vi "Image_Acquire_simulate.vi"(0 "Queue Ref in":T3, 1 "Acquire Time":i32=100, 3 "Image Out":T2, 5 "error in (no error)":errorcluster, 7 "Test Timing":bool) -> (6 "Loop Time Out":i64, 8 "error out":errorcluster)   [LabVIEW 2019]
uses:
  <vilib>/vision/Image Controls.llb/IMAQ Image.ctl
  <vilib>/userDefined/High Color/IMAQdx.ctl
  <vilib>/Platform/TimedLoop/XDataNode/timing_clust.ctl
  <vilib>/Platform/TimedLoop/XDataNode/nitl_modes.ctl
  <vilib>/Platform/TimedLoop/XDataNode/wakeup.ctl
  <vilib>/Platform/TimedLoop/XDataNode/XDataNode.xnode
  <vilib>/Platform/TimedLoop/XDataNode/XDNodeRunTimeDep.lvlib
panel:
  in  "Session In":T1
  out "Global End Time":i64
  out "Iteration Duration":i64
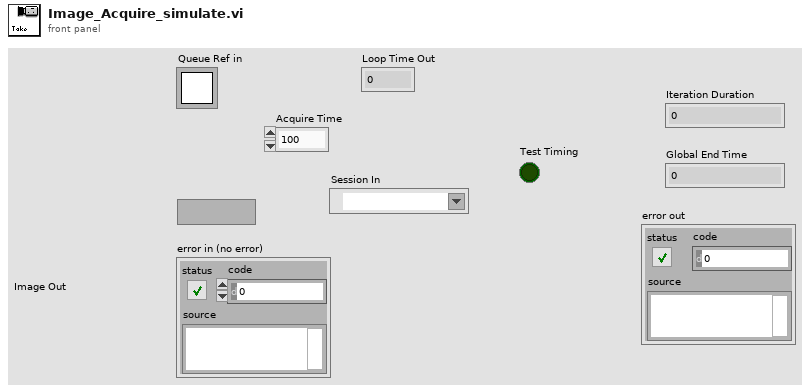
[diagram p1: front panel]
types:
  T1 = typedef "IMAQdx.ctl" = refnum<k21>
  T2 = typedef "IMAQ Image.ctl" = refnum<image>
  T3 = typedef "Queue RefNum" = refnum<k1>
  T4 = typedef "XDNodeRunTimeDep.lvlib/timing_clust.ctl" = cluster{"Expected End [f-1]":u64, "Actual End [f-1]":u64, "Finished Late? [f-1]":bool, "Expected End [i-1]":u64, "Actual End [i-1]":u64, "Finished Late? [i-1]":bool, "Expected Start [i]":u64, "Actual Start [i]":u64, "Expected Start [f]":u64, "Actual Start [f]":u64, "Source Name":string, "Structure Name":string, "Period":i64, "Deadline":i64, "Offset":i64, "Start":i64, "Priority":i32, "Timeout":i32, "Mode":T5, "Wakeup Reason":T6, "Error":errorcluster, "Source Type":string, "Secondary Source Type":string, "Global End Time":u64, "Global Start Time":u64, "Frame Duration":u64, "Iteration Duration":u64, "Assigned CPU":i32, "I/O Scan Engine Mode":u32}
  T5 = typedef "XDNodeRunTimeDep.lvlib/nitl_modes.ctl" = enum32{"No Change", "Process missed periods, maintain original phase", "Discard missed periods, maintain original phase", "Process missed periods, ignore original phase", "Discard missed periods, ignore original phase"}
  T6 = typedef "XDNodeRunTimeDep.lvlib/wakeup.ctl" = enum32{"Normal", "Aborted", "Asynchronous wakeup", "Timing source error", "Timed loop error", "Timeout"}
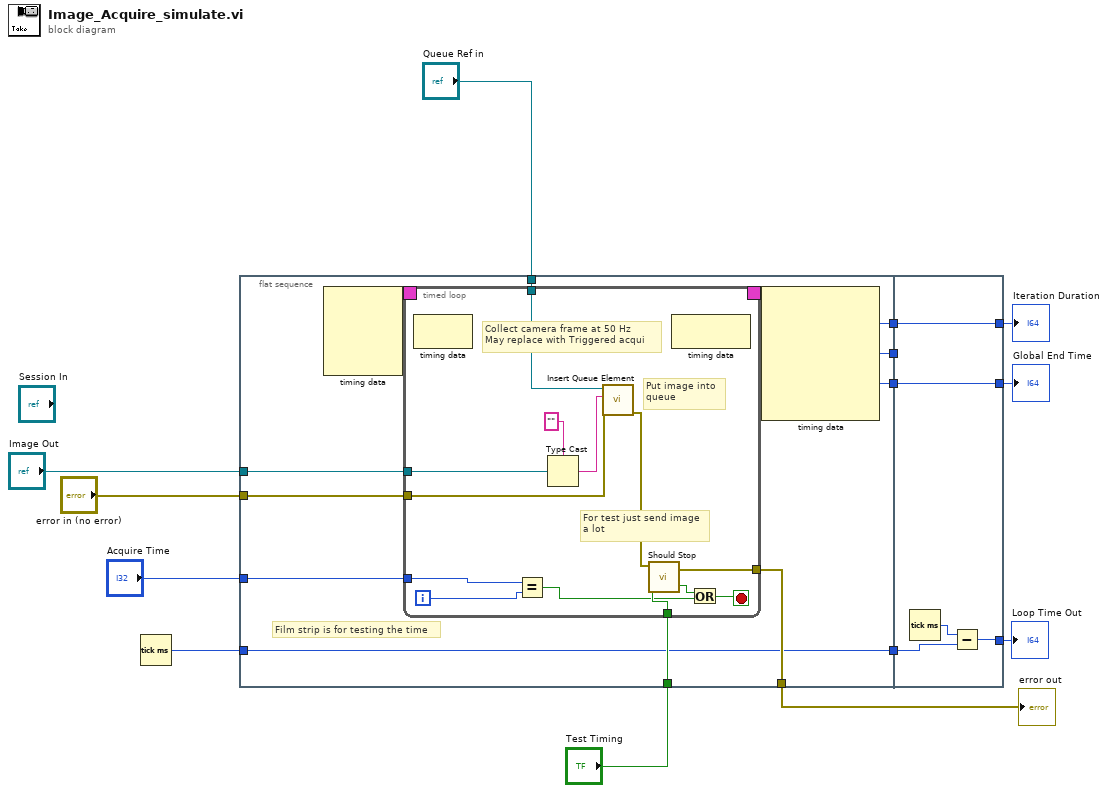
[diagram p0: block diagram]
diagram:
  n1 = Tick Count (ms)() -> (millisecond timer value=w1:u32)
  n2 = flat-sequence {
    tunnel: "error in (no error)" -> [w24]
    tunnel: "Image Out" -> [w23]
    tunnel: "Queue Ref in" -> [w22]
    tunnel: "Test Timing" -> [w21]
    tunnel: [w20] -> w10
    tunnel: [w19] -> w9
    tunnel: [w18] -> w7
    tunnel: [w17] -> w5
    tunnel: "Acquire Time" -> [w16]
    tunnel: [w15] -> w2
    tunnel: w1 -> [w15]
    tunnel: [w50] -> w8
    tunnel: w9 -> [w50]
    tunnel: [w51] -> w6
    tunnel: w7 -> [w51]
    tunnel: w5 -> [_]
    tunnel: [w47] -> w4
    tunnel: w2 -> [w49]
    frame #0 {
      # "Film strip is for testing the time"
      n3 = node-c288() -> (w26:T4)  [unwired: 4 in]
      n4 = timed-loop "Timed Loop" {
        timing: w26 -> [_]
        timing-out: [_] -> w25
        tunnel: w22 -> [w39]
        tunnel: [w37] -> w20
        tunnel: w24 -> [w30]
        tunnel: w23 -> [w36]
        tunnel: w21 -> [w33]
        tunnel: w16 -> [w32]
        i -> [w31]
        stop <- w28 stop-if-true
        # "Put image into\nqueue"
        # "For test just send image\na lot"
        # "Collect camera frame at 50 Hz\nMay replace with Triggered acqui"
        n5 = node-c288() -> ()  [unwired: 1 in, 1 out]
        n6 = Equal?(x=w32, y=w31) -> (x = y?=w27:bool)
        n7 = Type Cast(type="", x=w36) -> (*(type *) &x=w34:string)
        n8 = call <vilib>:"Insert Queue Element.vi"("error in (no error)"=w30, "queue element"=w34, "queue"=w39) -> ("error out"=w38:errorcluster)  [unwired: 4 in, 2 out]
        n9 = call "Should Stop.vi"("error in 1"=w38, "Look at Stop Button"=w33) -> ("error out"=w37:errorcluster, "Stop"=w29:bool)  [unwired: 3 in]
        n10 = node-c288() -> ()  [unwired: 1 in, 1 out]
        n11 = Or(x=w29, y=w27) -> (x .or. y?=w28:bool)
      }
      n12 = node-c288(w25) -> (w19:i64, w17:i64, w18:i64)  [unwired: 4 out]
    }
    frame #1 {
      n13 = Tick Count (ms)() -> (millisecond timer value=w48:u32)
      n14 = Subtract(x=w48, y=w49) -> (x-y=w47:u32)
    }
  }
  "Loop Time Out" <- w4
  "error out" <- w10
  "Iteration Duration" <- w8
  "Global End Time" <- w6
